vi "GetFirstNewErrorCode.vi"(8 "error in (no error)":errorcluster, 10 "LibraryName":string, 11 "Connection in":refnum<class "Connection.lvclass">) -> (0 "error out":errorcluster, 1 "Valid":bool, 2 "NewErrorCode":i32, 3 "Connection out":refnum<class "Connection.lvclass">)   [LabVIEW 2018, in "ErrorDefinitionSQLite.lvclass"]
uses:
  ErrorDefinitionSQLite.lvclass
  <vilib>/drjdpowell/SQLite Library/SQL Connection/Connection.lvclass
  <vilib>/drjdpowell/SQLite Library/SQL Connection/Execute SQL.vi
  <vilib>/drjdpowell/SQLite Library/SQLite.lvlib
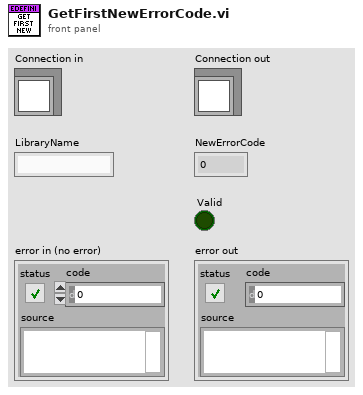
[diagram p1: front panel]
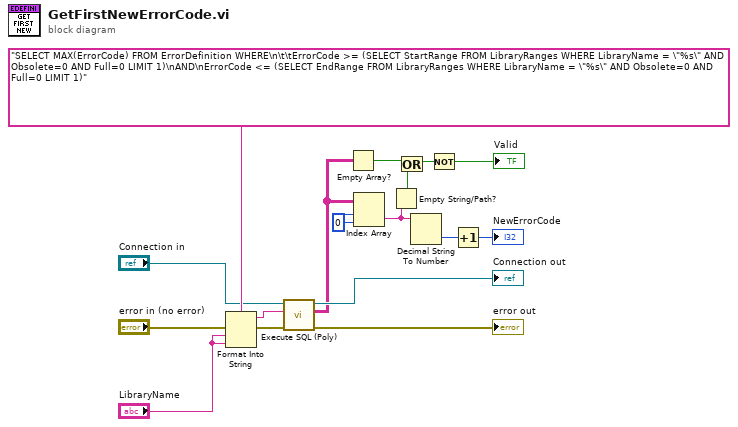
[diagram p0: block diagram]
diagram:
  w10 = 0 ("disabled index (col)")
  n1 = Format Into String(format string="SELECT MAX(ErrorCode) FROM ErrorDefinition WHERE\n\t\tErrorCode >= (SELECT StartRange FROM LibraryRanges WHERE LibraryName = \"%s\" AND Obsolete=0 AND Full=0 LIMIT 1)\nAND\nErrorCode <= (SELECT EndRange FROM LibraryRanges WHERE LibraryName = \"%s\" AND Obsolete=0 AND Full=0 LIMIT 1)" ("SQL"), error in="error in (no error)", "LibraryName", "LibraryName") -> (resulting string=w11:string, error out=w13:errorcluster)  [unwired: 1 in]
  n2 = call-poly <vilib>:"Execute SQL (Poly).vi"("error in (no error)"=w13, "SQL"=w11, "SQLite Connection in"="Connection in") -> ("error out"=→"error out":errorcluster, "Result Set"=w7:string[][], "SQLite Connection"=→"Connection out":refnum<class "Connection.lvclass">)  [unwired: 5 in, 1 out]
  n3 = Empty Array?(array=w7) -> (empty?=w6:bool)
  n4 = Index Array(array=w7, index (row)=w10, index (col)=w10) -> (element=w3:string)
  n5 = Empty String/Path?(string/path=w3) -> (empty?=w1:bool)
  n6 = Or(x=w6, y=w1) -> (x .or. y?=w2:bool)
  n7 = Decimal String To Number(string=w3) -> (number=w8:i32)  [unwired: 2 in, 1 out]
  n8 = Not(x=w2) -> (.not. x?=→"Valid":bool)
  n9 = Increment(x=w8) -> (x+1=→"NewErrorCode":i32)
